vi "CLC_GEN3_L2_InPhaseCal_mW_BaseOnly_L&S.vi"() -> ()   [LabVIEW 2023, in "Clover_Cell.lvlib"]
uses:
  Clover_Cell.lvlib
  lib/ELTA/ELTA.lvlib
  lib/R_S/R_S.lvlib
  lib/LitePoints/LitePoints.lvlib
panel:
  in  "Base_Gain":i32
  in  "Base_Phase":i32
  in  "Base_Ch":i32
  in  "Daul_Ch_Phase_Sweep":bool
  in  "SweepSwitch?":u16(ring) items=["NoSweep(Single)", "Sweep"]
  in  "SweepMode":u16(ring) items=["Phase", "Gain"]
  in  "Method":u16(ring)=1 items=["dBm"=1, "mW"=2]
  in  "Polarity":u16(ring) items=["H", "V"]
  in  "Spectrum_VISA":refnum<visa-resource-name>="TCPIP0::192.168.100.230::inst0::INSTR"
  in  "CenterFreq(GHz)":dbl=28.0
  in  "AvgTimes":i32=3
  in  "Single_Ch_Phase_Sweep":bool
  in  "TRXmode":u16(ring)=1 items=["Rx"=2, "Tx"=1]
  out "GainStep":i32=63
  out "PhaseStep":i32=63
  out "Channel":i32=63
  out "Total mW":dbl format="%.7f"
  out "Total dBm":dbl format="%.7f"
  out "Ref. mW":dbl format="%.7f"
  out "Ref. dBm":dbl format="%.7f"
  out "Main mW":dbl format="%.7f"
  out "Main dBm":dbl format="%.7f"
  out "Data":dbl[][](array[numeric])
  out "FileNAME_Single":string
  out "Spectrum Analyzer":dbl[](graph)
  out "CurrentData":dbl[](array[numeric])
  out "Duration":dbl
  out "TotalTime":dbl format="%.2f"
  out "StopTime":timestamp=timestamp(3663835912.033212 s since 1904-01-01)
  out "FileNAME_Dual":string
  out "StartTime":timestamp=timestamp(3663835741.875155 s since 1904-01-01)
  out "TX/RX":u16=1
  out "error out":errorcluster
  out "output cluster":T1={"address"="192.168.100.111", "remote port or service name"=5025, "timeout ms (60000)"=10000}
  out "Operating \nChannel(s)":bool[][](array[boolean])
  out "OK?":bool
  # "TMYTEK_CLC_JIO_One_Panel_Phase_Calibration"
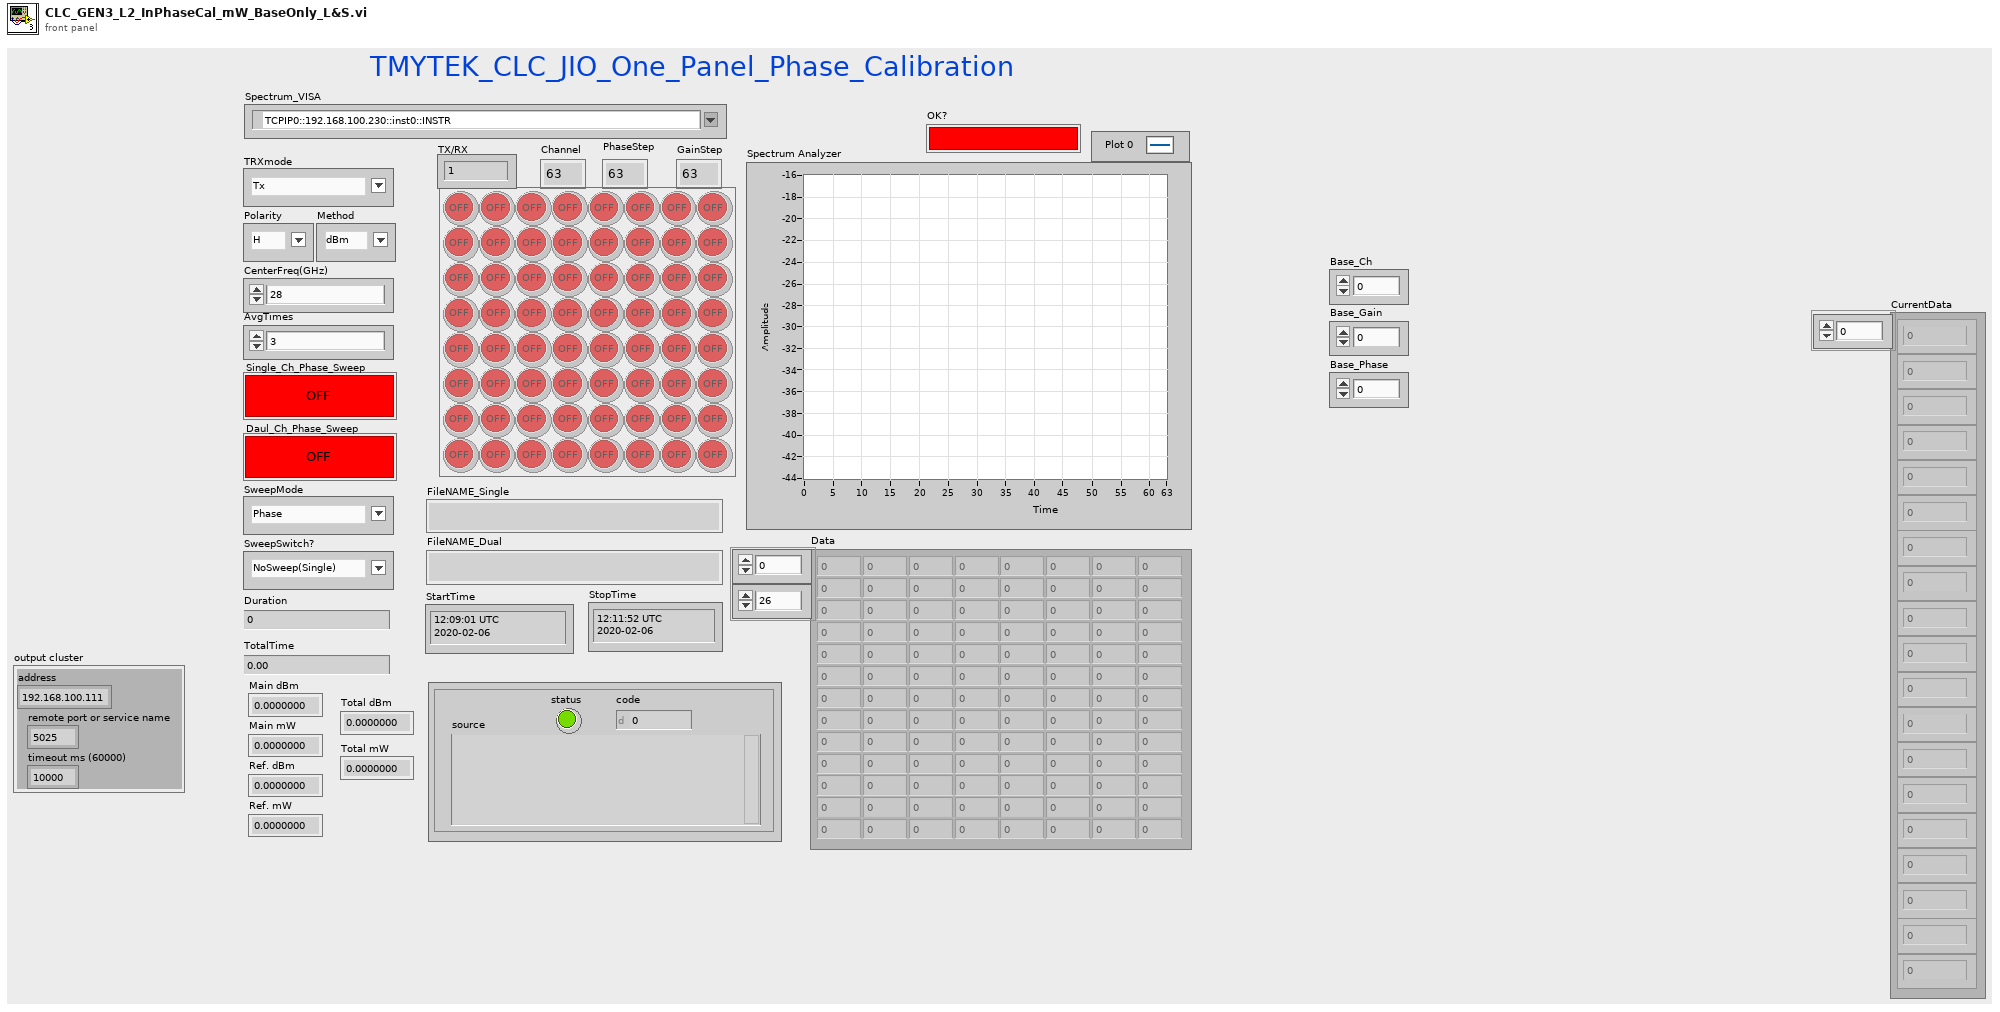
[diagram p1: front panel]
types:
  T1 = cluster{"address":string, "remote port or service name":u16, "timeout ms (60000)":i32}
  T2 = cluster{"Mode":u16, "Polarity":u16, "CH_ON/OFF":u16, "Channel":i32, "Gain":i32, "Phase":i32}
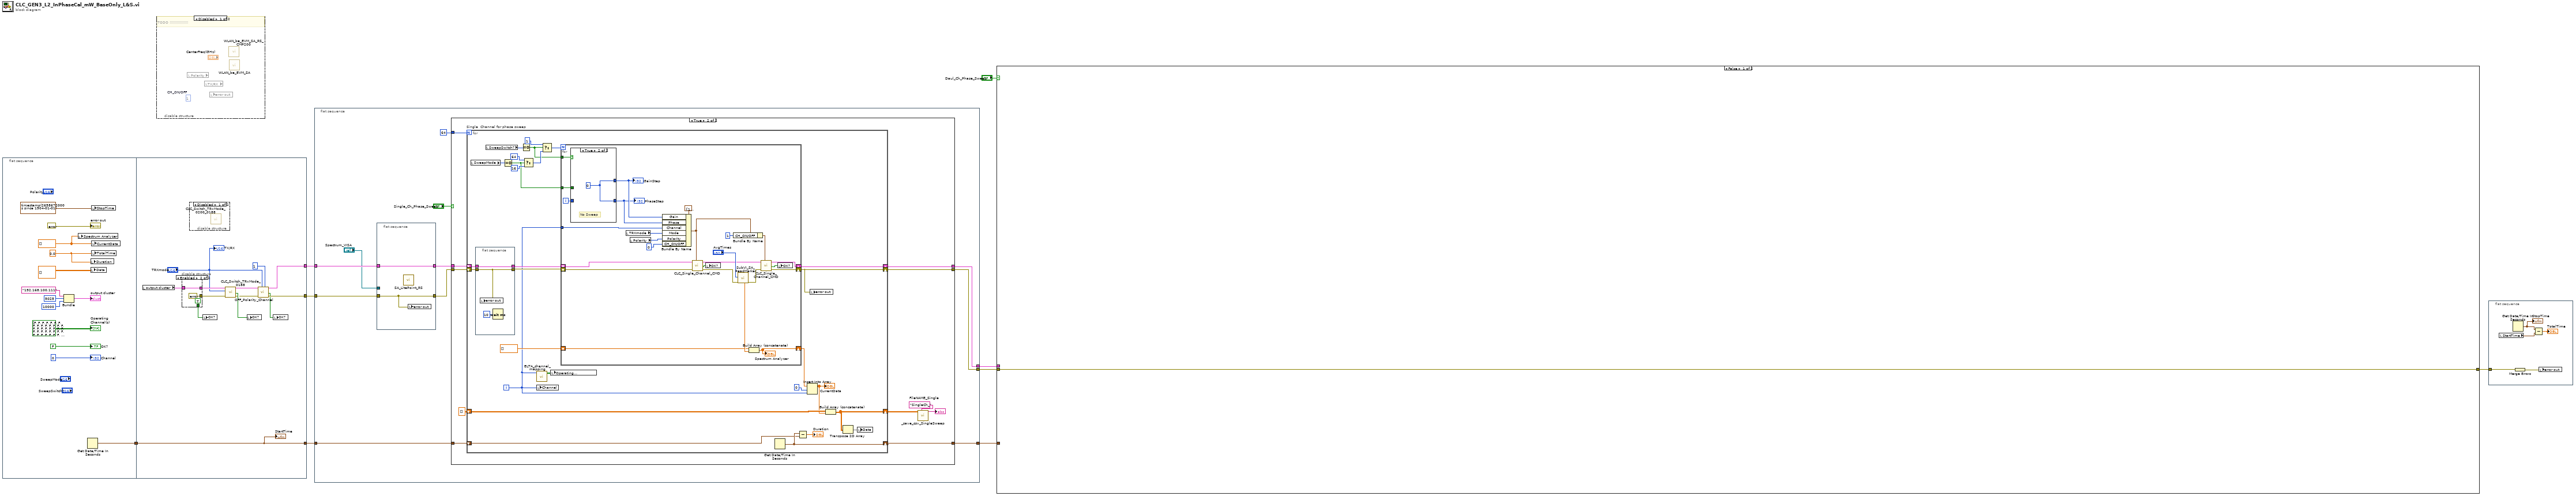
[diagram p0: block diagram]
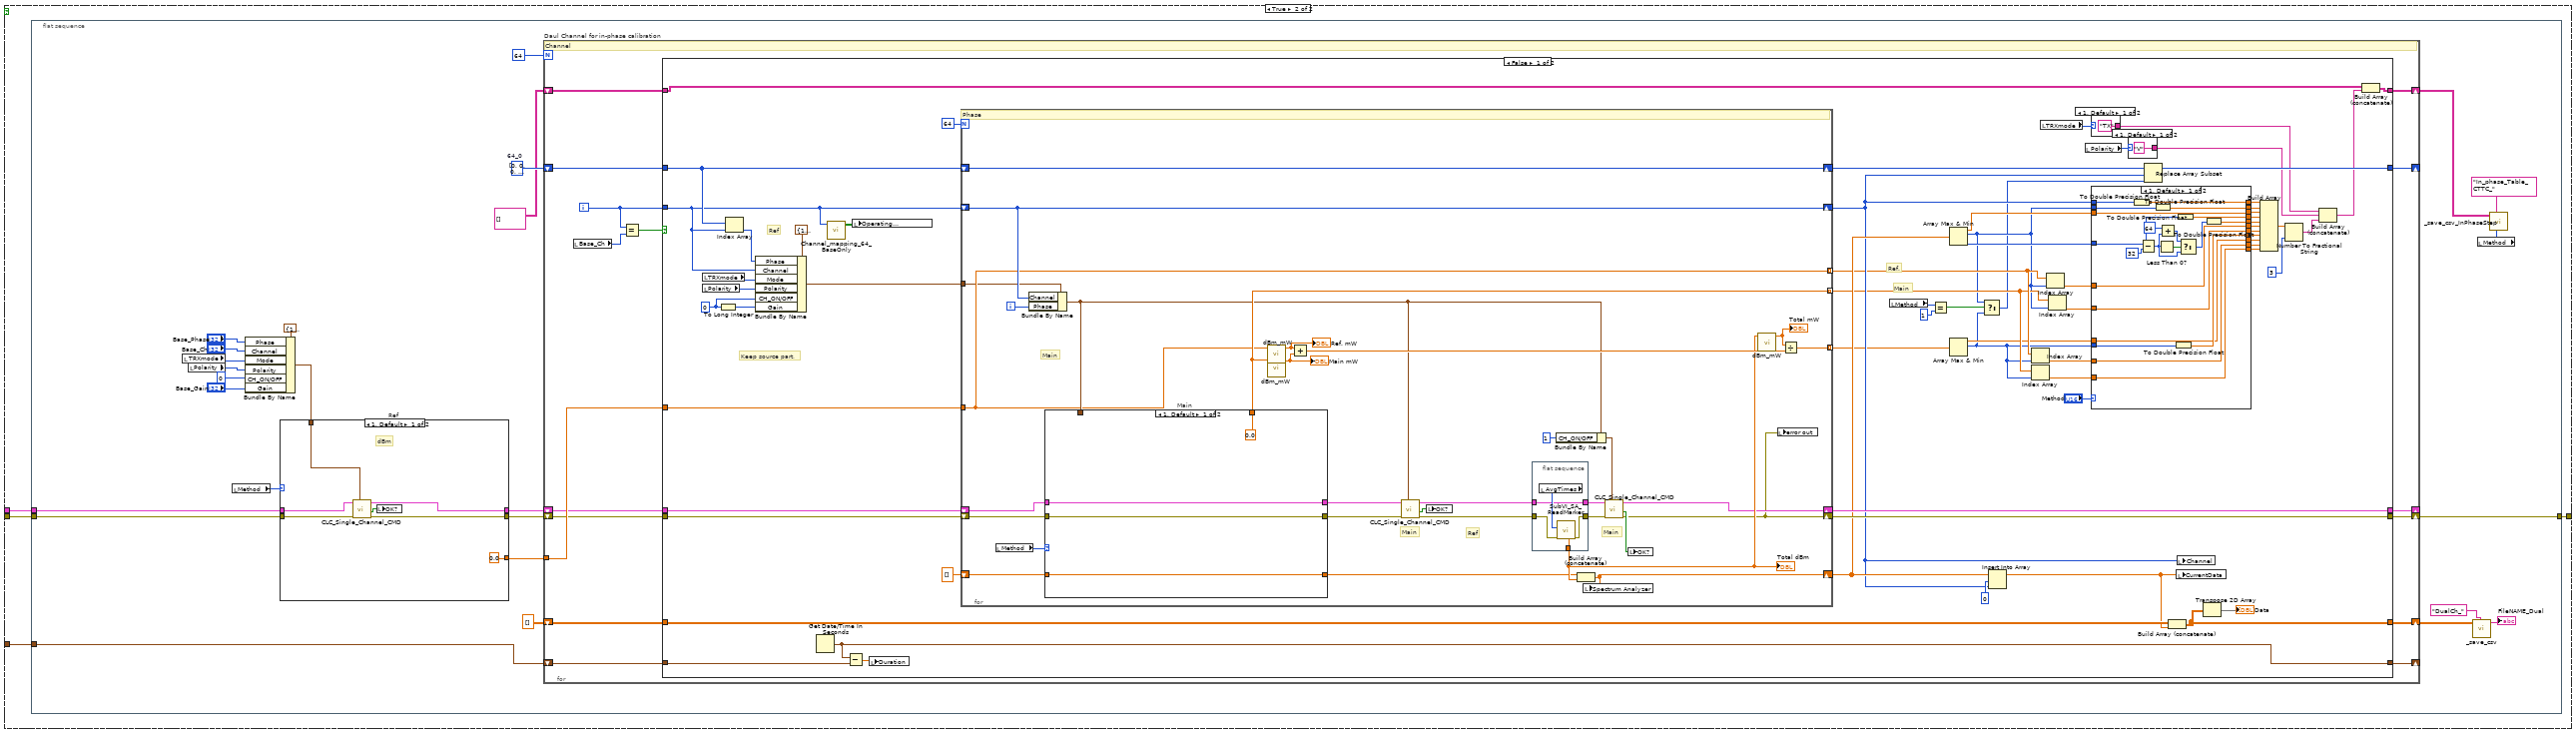
[diagram p3: hidden frame]
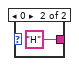
[diagram p4: hidden frame]
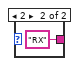
[diagram p5: hidden frame]
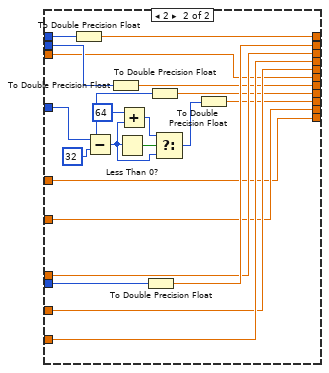
[diagram p6: hidden frame]
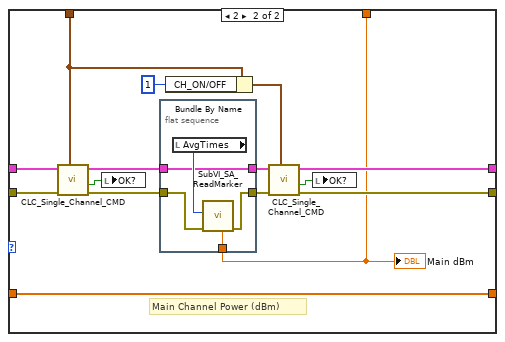
[diagram p7: hidden frame]
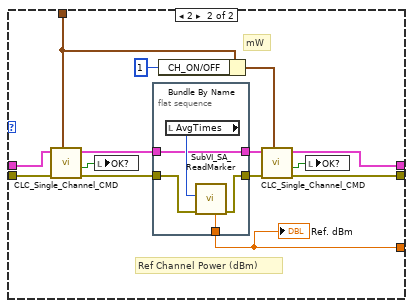
[diagram p9: hidden frame]
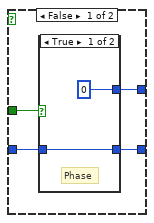
[diagram p11: hidden frame]
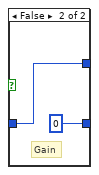
[diagram p12: hidden frame]
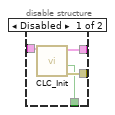
[diagram p14: hidden frame]
diagram:
  n1 = flat-sequence {
    tunnel: [w10] -> w9
    tunnel: w9 -> [w25]
    tunnel: [w27] -> w2
    tunnel: [w30] -> w3
    tunnel: [w25] -> w8
    frame #0 {
      w14 = dbl[] []
      w17 = 0.0 ("TotalTime")
      n2 = Bundle("address"="192.168.100.111", "remote port or service name"=u16 5025, "timeout ms (60000)"=10000) -> (→"output cluster":T1)  [unwired: 1 in]
      n3 = local write "Spectrum Analyzer"(w14) -> ()
      n4 = Get Date/Time In Seconds() -> (seconds since 1Jan1904=w10:timestamp)
      n5 = local write "Duration"(w17) -> ()
      n6 = local write "Data"(dbl[][] []) -> ()
      n7 = local write "StopTime"(timestamp(2658672000.001 s since 1904-01-01) ("StopTime")) -> ()
      n8 = local write "CurrentData"(w14) -> ()
      n9 = local write "TotalTime"(w17) -> ()
      "error out" <- errorcluster {"status"=FALSE, "code"=0, "source"=""} ("error out")
      "Operating \nChannel(s)" <- bool[][] [[FALSE, FALSE, FALSE, FALSE, FALSE, FALSE, FALSE, FALSE], [FALSE, FALSE, FALSE, FALSE, FALSE, FALSE, FALSE, FALSE], [FALSE, FALSE, FALSE, FALSE, FALSE, FALSE, FALSE, FALSE], [FALSE, FALSE, FALSE, FALSE, FALSE, FALSE, FALSE, FALSE], [FALSE, FALSE, FALSE, FALSE, FALSE, FALSE, FALSE, FALSE], [FALSE, FALSE, FALSE, FALSE, FALSE, FALSE, FALSE, FALSE], [FALSE, FALSE, FALSE, FALSE, FALSE, FALSE, FALSE, FALSE], [FALSE, FALSE, FALSE, FALSE, FALSE, FALSE, FALSE, FALSE]] ("Operating \nChannel(s)")
      "Channel" <- 0 ("Channel")
      "OK?" <- FALSE ("OK?")
    }
    frame #1 {
      n10 = local read "output cluster"() -> (w35:T1)
      n11 = disable-structure shown="Enabled" {
        disable-tunnel: w35 -> [w39 w42]
        disable-tunnel: [w38 w42] -> w34
        disable-tunnel: [w37 errorcluster {"status"=FALSE, "code"=0, "source"=""} ("error in (no error)")] -> w32
        disable-tunnel: [w36 TRUE ("OK?")] -> w26
        frame Disabled {
          n12 = call "CLC_Init.vi"("TCPIPin"=w39) -> ("error out"=w37:errorcluster, "Status"=w36:bool, "TCPIPin 2"=w38:T1)  [unwired: 8 in]
        }
        frame Enabled {
        }
      }
      n13 = disable-structure shown="Disabled" {
        frame Disabled {
          n14 = call "CLC_Switch_TRxMode_0200_0188.vi"() -> ()  [unwired: 9 in, 3 out]
        }
        frame Enabled {
        }
      }
      n15 = local write "OK?"(w26) -> ()
      n16 = call "CLC_Switch_TRxMode_0188.vi"("error in (no error)"=w32, "Text Ring"="TRXmode", "TCPIPin"=w34) -> ("error out"=w31:errorcluster, "OK?"=w33:bool, "TCPIPin 2"=w29:T1)  [unwired: 6 in]
      n17 = local write "OK?"(w33) -> ()
      n18 = call "OFF_Polarity_Channel.vi"("CH_ON:0/OFF:1"=u16 1, "Mode"="TRXmode", "error in"=w31, "TCPIPin"=w29) -> ("error out"=w30:errorcluster, "OK?"=w28:bool, "TCPIPout"=w27:T1)  [unwired: 5 in]
      n19 = local write "OK?"(w28) -> ()
      "StartTime" <- w25
      "TX/RX" <- "TRXmode"
    }
  }
  n20 = disable-structure shown="Disabled" {
    frame Disabled {
      (unwired) u16 1  # CH_ON/OFF
      # "TODO !!!!!!!!!!!!!!!!"
      n21 = local read "Polarity"() -> ()  [unwired: 1 out]
      n22 = local read "TX/RX"() -> ()  [unwired: 1 out]
      n23 = local read "error out"() -> ()  [unwired: 1 in]
      n24 = call "WLAN_be_EVM_SA_RS_CMP200.vi"() -> ()  [unwired: 8 in, 4 out]
      n25 = call "WLAN_be_EVM_SA.vi"() -> ()  [unwired: 8 in, 4 out]
    }
    frame Enabled {
    }
  }
  n26 = flat-sequence {
    tunnel: w8 -> [w52]
    tunnel: [w51] -> w7
    tunnel: [w50] -> w6
    tunnel: [w49] -> w4
    tunnel: w3 -> [w48]
    tunnel: w2 -> [w46]
    frame #0 {
      n27 = flat-sequence {
        tunnel: w48 -> [w134]
        tunnel: [w134] -> w47
        tunnel: w46 -> [w133]
        tunnel: "Spectrum_VISA" -> [_]
        tunnel: [w133] -> w44
        frame #0 {
          n28 = call "SA_LitePoint_RS.vi"() -> ()  [unwired: 12 in]
          n29 = local write "error out"(w134) -> ()
        }
      }
      n30 = case shown="True" "Single_Ch_Phase_Sweep" {
        tunnel: 64 -> [_ w67]
        tunnel: w52 -> [w54 w66]
        tunnel: [w55 w65] -> w51
        tunnel: [w56 w64] -> w50
        tunnel: [w54 w63] -> w49
        tunnel: w47 -> [w55 w62]
        tunnel: w44 -> [w56 w61]
        frame False {
        }
        frame True {
          n31 = for "Single  Channel for phase sweep" {
            N: w67 -> [_]
            shift-right: [w94] -> w64
            shift-left: w61 -> [w81]
            shift-right: [w90] -> w65
            shift-left: w62 -> [w83]
            shift-right: [w88] -> w58
            shift-left: dbl[][] [] -> [w89]
            shift-right: [w92] -> w63
            shift-left: w66 -> [w91]
            i -> [w68]
            n32 = local read "SweepMode"() -> (w77:u16)
            n33 = flat-sequence {
              tunnel: [w95] -> w80
              tunnel: w83 -> [w96]
              tunnel: [w96] -> w82
              tunnel: w81 -> [w95]
              frame #0 {
                n34 = local write "error out"(w96) -> ()
                n35 = Wait (ms)(milliseconds to wait=u32 10) -> ()  [unwired: 1 out]
              }
            }
            n36 = local read "SweepSwitch?"() -> (w76:u16)
            n37 = Equal To 0?(x=w77) -> (x = 0?=w69:bool)
            n38 = Equal To 0?(x=w76) -> (x = 0?=w70:bool)
            n39 = Select(t=64, s=w69, f=16) -> (s? t:f=w71:i32)
            n40 = local write "Channel"(w68) -> ()
            n41 = call "ELTA_channel_mapping.vi"("Ch_1_ref"=w68) -> ("Operating \nChannel(s)"=w78:bool[][])  [unwired: 10 in]
            n42 = Select(t=1, s=w70, f=w71) -> (s? t:f=w74:i32)
            n43 = local write "Operating \nChannel(s)"(w78) -> ()
            n44 = for {
              N: w74 -> [_]
              shift-right: [w107] -> w94
              shift-left: w80 -> [w117]
              shift-right: [w109] -> w90
              shift-left: w82 -> [w119]
              shift-right: [w120] -> w87
              shift-left: dbl[] [] -> [w121]
              tunnel: w68 -> [w114]
              tunnel: w70 -> [w102]
              tunnel: w69 -> [w99]
              i -> [w98]
              n45 = case shown="True" w102 {
                tunnel: [w124 w132] -> w101
                tunnel: [w125 w132] -> w100
                tunnel: w99 -> [w127 _]
                tunnel: w98 -> [w126 _]
                frame False {
                  n46 = case shown="True" w127 {
                    tunnel: w126 -> [w129 w130]
                    tunnel: [w129 0] -> w125
                    tunnel: [0 w130] -> w124
                    frame True {
                      # "Phase"
                    }
                    frame False {
                      # "Gain"
                    }
                  }
                }
                frame True {
                  w132 = 0
                  # "No Sweep"
                }
              }
              "PhaseStep" <- w100
              "GainStep" <- w101
              n47 = local read "TRXmode"() -> (w113:u16)
              n48 = local read "Polarity"() -> (w112:u16)
              n49 = Bundle By Name(cluster=T2 {"Mode"=1, "Polarity"=1, "CH_ON/OFF"=1, "Channel"=0, "Gain"=0, "Phase"=0} ("Channel params"), "Gain"=w101, "Phase"=w100, "Channel"=w114, "Mode"=w113, "Polarity"=w112, "CH_ON/OFF"=u16 0) -> (w106:T2)
              n50 = call "CLC_Single_Channel_CMD.vi"("Channel params"=w106, "error in"=w119, "TCPIPin"=w117) -> ("error out"=w118:errorcluster, "OK?"=w115:bool, "TCPIPout"=w108:T1)  [unwired: 6 in]
              n51 = local write "OK?"(w115) -> ()
              n52 = Bundle By Name(cluster=w106, "CH_ON/OFF"=u16 1) -> (w104:T2)
              n53 = call "SubVI_SA_ReadMarker.vi"("error in (no error)"=w118, "AvgTimes"="AvgTimes") -> ("error out"=w110:errorcluster, "Marker Power"=w122:dbl)  [unwired: 6 in, 2 out]
              n54 = Build Array (concatenate)(w121, w122) -> (w120:dbl[])
              "Spectrum Analyzer" <- w120
              n55 = call "CLC_Single_Channel_CMD.vi"("Channel params"=w104, "error in"=w110, "TCPIPin"=w108) -> ("error out"=w109:errorcluster, "OK?"=w103:bool, "TCPIPout"=w107:T1)  [unwired: 6 in]
              n56 = local write "OK?"(w103) -> ()
            }
            n57 = Get Date/Time In Seconds() -> (seconds since 1Jan1904=w92:timestamp)
            n58 = Subtract(x=w92, y=w91) -> (x-y=→"Duration":dbl)
            n59 = Insert Into Array(array=w87, index=0, new element=w68) -> (w85:dbl[])
            "CurrentData" <- w85
            n60 = local write "error out"(w90) -> ()
            n61 = Build Array (concatenate)(w89, w85) -> (w88:dbl[][])
            n62 = Transpose 2D Array(2D array=w88) -> (transposed array=w79:dbl[][])
            n63 = local write "Data"(w79) -> ()
          }
          n64 = call "_save_csv_SingleSweep.vi"("delimiter (\\t)"="SingleCh_" ("delimiter (\\t)"), "Data"=w58) -> ("FileName"=→"FileNAME_Single":string)  [unwired: 9 in]
        }
      }
    }
  }
  n65 = case shown="False" "Daul_Ch_Phase_Sweep" {
    tunnel: w7 -> [w135 w139]
    tunnel: w6 -> [_ w138]
    tunnel: [w135 w137] -> w5
    tunnel: w4 -> [_ w136]
    frame False {
    }
    frame True {
      n66 = flat-sequence {
        tunnel: w139 -> [w150]
        tunnel: w138 -> [w151]
        tunnel: [w164] -> w137
        tunnel: w136 -> [w163]
        frame #0 {
          w161 = i32[] [0, 0, 0, 0, 0, 0, 0, 0, 0, 0, 0, 0, 0, 0, 0, 0, 0, 0, 0, 0, 0, 0, 0, 0, 0, 0, 0, 0, 0, 0, 0, 0, 0, 0, 0, 0, 0, 0, 0, 0, 0, 0, 0, 0, 0, 0, 0, 0, 0, 0, 0, 0, 0, 0, 0, 0, 0, 0, 0, 0, 0, 0, 0, 0]  # 64_0
          n67 = local read "TRXmode"() -> (w147:u16)
          n68 = local read "Polarity"() -> (w148:u16)
          n69 = local read "Method"() -> (w155:u16)
          n70 = Bundle By Name(cluster=T2 {"Mode"=1, "Polarity"=1, "CH_ON/OFF"=1, "Channel"=0, "Gain"=0, "Phase"=0} ("Channel params"), "Phase"="Base_Phase", "Channel"="Base_Ch", "Mode"=w147, "Polarity"=w148, "CH_ON/OFF"=u16 0, "Gain"="Base_Gain") -> (w145:T2)
          n71 = case "Ref" shown="1, Default" w155 {
            tunnel: w150 -> [w363 w373]
            tunnel: [w366 w372] -> w153
            tunnel: w151 -> [w364 w371]
            tunnel: [w365 w370] -> w152
            tunnel: [0.0 ("Marker Response") w369] -> w154
            tunnel: w145 -> [w362 w368]
            frame 1, Default {
              # "dBm"
              n72 = call "CLC_Single_Channel_CMD.vi"("Channel params"=w362, "error in"=w363, "TCPIPin"=w364) -> ("error out"=w366:errorcluster, "OK?"=w361:bool, "TCPIPout"=w365:T1)  [unwired: 6 in]
              n73 = local write "OK?"(w361) -> ()
            }
            frame 2 {
              # "mW"
              # "Ref Channel Power (dBm)"
              n74 = call "CLC_Single_Channel_CMD.vi"("Channel params"=w368, "error in"=w373, "TCPIPin"=w371) -> ("error out"=w380:errorcluster, "OK?"=w381:bool, "TCPIPout"=w379:T1)  [unwired: 6 in]
              n75 = local write "OK?"(w381) -> ()
              n76 = flat-sequence {
                tunnel: [w385] -> w369
                tunnel: w380 -> [w384]
                tunnel: [w383] -> w375
                tunnel: w379 -> [w383]
                tunnel: [w382] -> w376
                frame #0 {
                  n77 = local read "AvgTimes"() -> (w386:i32)
                  n78 = call "SubVI_SA_ReadMarker.vi"("error in (no error)"=w384, "AvgTimes"=w386) -> ("error out"=w382:errorcluster, "Marker Power"=w385:dbl)  [unwired: 6 in, 2 out]
                }
              }
              n79 = Bundle By Name(cluster=w368, "CH_ON/OFF"=u16 1) -> (w377:T2)
              n80 = call "CLC_Single_Channel_CMD.vi"("Channel params"=w377, "error in"=w376, "TCPIPin"=w375) -> ("error out"=w372:errorcluster, "OK?"=w378:bool, "TCPIPout"=w370:T1)  [unwired: 6 in]
              n81 = local write "OK?"(w378) -> ()
              "Ref. dBm" <- w369
            }
          }
          n82 = for "Daul Channel for in-phase calibration" {
            N: 64 -> [_]
            shift-right: [w181] -> _
            shift-left: w152 -> [w171]
            shift-right: [w180] -> w164
            shift-left: w153 -> [w170]
            shift-right: [w176] -> w157
            shift-left: dbl[][] [] -> [w177]
            shift-right: [w179] -> _
            shift-left: w163 -> [w178]
            shift-right: [w175] -> _
            shift-left: w161 -> [w174]
            tunnel: w154 -> [w172]
            shift-right: [w173] -> w141
            shift-left: string[][] [] -> [w166]
            i -> [w168]
            # "Channel"
            n83 = local read "Base_Ch"() -> (w169:i32)
            n84 = Equal?(x=w168, y=w169) -> (x = y?=w167:bool)
            n85 = case shown="False" w167 {
              tunnel: [w248 w359] -> w181
              tunnel: [w246 w358] -> w180
              tunnel: [w245 w356] -> w179
              tunnel: w178 -> [w244 w356]
              tunnel: w177 -> [w242 w357]
              tunnel: [w241 w357] -> w176
              tunnel: [w235 w360] -> w175
              tunnel: w174 -> [w217 w360]
              tunnel: [w183 w355] -> w173
              tunnel: w172 -> [w188 _]
              tunnel: w171 -> [w187 w359]
              tunnel: w170 -> [w186 w358]
              tunnel: w168 -> [w185 _]
              tunnel: w166 -> [w182 w355]
              frame False {
                w219 = u16 0 ("CH_ON/OFF")
                # "Keep source part,"
                # "Main"
                # "Ref."
                # "Ref"
                n86 = local read "TRXmode"() -> (w221:u16)
                n87 = local read "Polarity"() -> (w220:u16)
                n88 = To Long Integer(number=w219) -> (32bit integer=w218:i32)
                n89 = Index Array(array=w217, index=w185) -> (element=w216:i32)
                n90 = Bundle By Name(cluster=T2 {"Mode"=1, "Polarity"=1, "CH_ON/OFF"=1, "Channel"=0, "Gain"=0, "Phase"=0} ("Channel params"), "Phase"=w216, "Channel"=w185, "Mode"=w221, "Polarity"=w220, "CH_ON/OFF"=w219, "Gain"=w218) -> (w184:T2)
                n91 = Get Date/Time In Seconds() -> (seconds since 1Jan1904=w245:timestamp)
                n92 = call "Channel_mapping_64_BaseOnly.vi"("Channel IN"=w185) -> ("Operating \nChannel(s)"=w223:bool[][])  [unwired: 10 in]
                n93 = Subtract(x=w245, y=w244) -> (x-y=w243:dbl)
                n94 = local write "Operating \nChannel(s)"(w223) -> ()
                n95 = local write "Duration"(w243) -> ()
                n96 = for {
                  N: 64 -> [_]
                  shift-right: [w297] -> w248
                  shift-left: w187 -> [w307]
                  shift-right: [w296] -> w246
                  shift-left: w186 -> [w318]
                  shift-right: [w320] -> w236
                  shift-left: dbl[] [] -> [w309]
                  shift-right: [w324] -> w234
                  shift-left: w217 -> [w324]
                  shift-right: [w303] -> w233
                  shift-left: w185 -> [w303]
                  tunnel: [w300] -> w226 mode=indexing
                  tunnel: [w313] -> w225 mode=indexing
                  tunnel: [w314] -> w232 mode=indexing
                  tunnel: w188 -> [w300]
                  tunnel: w184 -> [w295]
                  i -> [w304]
                  # "Main"
                  # "Main"
                  # "Ref"
                  # "Main"
                  # "Phase"
                  n97 = local read "Method"() -> (w310:u16)
                  n98 = Bundle By Name(cluster=w295, "Channel"=w303, "Phase"=w304) -> (w302:T2)
                  n99 = case "Main" shown="1, Default" w310 {
                    tunnel: w318 -> [w327 w332]
                    tunnel: w307 -> [w328 w333]
                    tunnel: [w328 w336] -> w317
                    tunnel: [w327 w335] -> w316
                    tunnel: w302 -> [_ w334]
                    tunnel: [0.0 ("Marker Response") w330] -> w313
                    tunnel: w309 -> [w326 w331]
                    tunnel: [w326 w331] -> w308
                    frame 1, Default {
                    }
                    frame 2 {
                      # "Main Channel Power (dBm)"
                      n100 = call "CLC_Single_Channel_CMD.vi"("Channel params"=w334, "error in"=w332, "TCPIPin"=w333) -> ("error out"=w338:errorcluster, "OK?"=w337:bool, "TCPIPout"=w339:T1)  [unwired: 6 in]
                      n101 = local write "OK?"(w337) -> ()
                      n102 = flat-sequence {
                        tunnel: [w348] -> w330
                        tunnel: w338 -> [w347]
                        tunnel: [w346] -> w344
                        tunnel: w339 -> [w346]
                        tunnel: [w345] -> w343
                        frame #0 {
                          n103 = local read "AvgTimes"() -> (w349:i32)
                          n104 = call "SubVI_SA_ReadMarker.vi"("error in (no error)"=w347, "AvgTimes"=w349) -> ("error out"=w345:errorcluster, "Marker Power"=w348:dbl)  [unwired: 6 in, 2 out]
                        }
                      }
                      n105 = Bundle By Name(cluster=w334, "CH_ON/OFF"=u16 1) -> (w342:T2)
                      n106 = call "CLC_Single_Channel_CMD.vi"("Channel params"=w342, "error in"=w343, "TCPIPin"=w344) -> ("error out"=w335:errorcluster, "OK?"=w340:bool, "TCPIPout"=w336:T1)  [unwired: 6 in]
                      n107 = local write "OK?"(w340) -> ()
                      "Main dBm" <- w330
                    }
                  }
                  n108 = call "dBm_mW.vi"("dBm"=w300) -> ("mW"=w306:dbl)  [unwired: 10 in]
                  "Ref. mW" <- w306
                  n109 = call "dBm_mW.vi"("dBm"=w313) -> ("mW"=w305:dbl)  [unwired: 10 in]
                  "Main mW" <- w305
                  n110 = Add(x=w306, y=w305) -> (x+y=w315:dbl)
                  n111 = call "CLC_Single_Channel_CMD.vi"("Channel params"=w302, "error in"=w316, "TCPIPin"=w317) -> ("error out"=w298:errorcluster, "OK?"=w325:bool, "TCPIPout"=w299:T1)  [unwired: 6 in]
                  n112 = local write "OK?"(w325) -> ()
                  n113 = flat-sequence {
                    tunnel: [w353] -> w312
                    tunnel: w298 -> [w352]
                    tunnel: [w351] -> w323
                    tunnel: w299 -> [w351]
                    tunnel: [w350] -> w319
                    frame #0 {
                      n114 = local read "AvgTimes"() -> (w354:i32)
                      n115 = call "SubVI_SA_ReadMarker.vi"("error in (no error)"=w352, "AvgTimes"=w354) -> ("error out"=w350:errorcluster, "Marker Power"=w353:dbl)  [unwired: 6 in, 2 out]
                    }
                  }
                  n116 = Bundle By Name(cluster=w302, "CH_ON/OFF"=u16 1) -> (w321:T2)
                  n117 = Build Array (concatenate)(w308, w312) -> (w320:dbl[])
                  n118 = local write "Spectrum Analyzer"(w320) -> ()
                  n119 = call "CLC_Single_Channel_CMD.vi"("Channel params"=w321, "error in"=w319, "TCPIPin"=w323) -> ("error out"=w296:errorcluster, "OK?"=w322:bool, "TCPIPout"=w297:T1)  [unwired: 6 in]
                  n120 = local write "OK?"(w322) -> ()
                  n121 = call "dBm_mW.vi"("dBm"=w312) -> ("mW"=w311:dbl)  [unwired: 10 in]
                  "Total mW" <- w311
                  n122 = local write "error out"(w296) -> ()
                  n123 = Divide(x=w311, y=w315) -> (x/y=w314:dbl)
                  "Total dBm" <- w312
                }
                n124 = local read "Method"() -> (w203:u16)
                n125 = Equal?(x=w203, y=u16 1) -> (x = y?=w201:bool)
                n126 = Array Max & Min(array=w236) -> (max value=w213:dbl, max index (indices)=w200:i32, min index (indices)=w224:i32)  [unwired: 1 out]
                n127 = Array Max & Min(array=w232) -> (max value=w207:dbl, max index (indices)=w199:i32)  [unwired: 2 out]
                n128 = Select(t=w200, s=w201, f=w199) -> (s? t:f=w198:i32)
                n129 = Insert Into Array(array=w236, index=0, new element=w233) -> (w237:dbl[])
                n130 = Index Array(array=w226, index=w199) -> (element=w206:dbl)
                n131 = Index Array(array=w225, index=w199) -> (element=w205:dbl)
                n132 = local read "TRXmode"() -> (w194:u16)
                n133 = Index Array(array=w226, index=w200) -> (element=w211:dbl)
                n134 = Index Array(array=w225, index=w200) -> (element=w210:dbl)
                n135 = local read "Polarity"() -> (w193:u16)
                n136 = case shown="1, Default" w194 {
                  tunnel: ["TX" "RX"] -> w190
                  frame 1, Default {
                  }
                  frame 2 {
                  }
                }
                n137 = case shown="1, Default" "Method" {
                  tunnel: w233 -> [w267 w288]
                  tunnel: [w253 w282] -> w231
                  tunnel: [w266 w281] -> w230
                  tunnel: [w265 w280] -> w229
                  tunnel: [w264 w284] -> w228
                  tunnel: [w263 w277] -> w227
                  tunnel: w224 -> [w262 w287]
                  tunnel: w199 -> [w261 w286]
                  tunnel: w200 -> [w260 w285]
                  tunnel: w213 -> [w253 w279]
                  tunnel: [w254 w283] -> w214
                  tunnel: [w259 w279] -> w212
                  tunnel: w211 -> [w259 w274]
                  tunnel: w210 -> [w258 w275]
                  tunnel: [w258 w278] -> w209
                  tunnel: [w257 w276] -> w208
                  tunnel: w207 -> [w257 w282]
                  tunnel: w206 -> [w256 w280]
                  tunnel: w205 -> [w255 w281]
                  tunnel: [w255 w274] -> w204
                  tunnel: [w256 w275] -> w197
                  frame 1, Default {
                    n138 = To Double Precision Float(number=w267) -> (double precision float=w264:dbl)
                    n139 = Subtract(x=w262, y=32) -> (x-y=w269:i32)
                    n140 = To Double Precision Float(number=w260) -> (double precision float=w254:dbl)
                    n141 = Less Than 0?(x=w269) -> (x < 0?=w272:bool)
                    n142 = Add(x=64, y=w269) -> (x+y=w270:i32)
                    n143 = To Double Precision Float(number=w261) -> (double precision float=w263:dbl)
                    n144 = To Double Precision Float(number=w262) -> (double precision float=w266:dbl)
                    n145 = Select(t=w270, s=w272, f=w269) -> (s? t:f=w268:i32)
                    n146 = To Double Precision Float(number=w268) -> (double precision float=w265:dbl)
                  }
                  frame 2 {
                    n147 = To Double Precision Float(number=w288) -> (double precision float=w284:dbl)
                    n148 = Subtract(x=w287, y=32) -> (x-y=w290:i32)
                    n149 = To Double Precision Float(number=w285) -> (double precision float=w278:dbl)
                    n150 = Less Than 0?(x=w290) -> (x < 0?=w293:bool)
                    n151 = Add(x=64, y=w290) -> (x+y=w291:i32)
                    n152 = To Double Precision Float(number=w286) -> (double precision float=w283:dbl)
                    n153 = To Double Precision Float(number=w287) -> (double precision float=w277:dbl)
                    n154 = Select(t=w291, s=w293, f=w290) -> (s? t:f=w289:i32)
                    n155 = To Double Precision Float(number=w289) -> (double precision float=w276:dbl)
                  }
                }
                n156 = case shown="1, Default" w193 {
                  tunnel: ["V" "H"] -> w191
                  frame 1, Default {
                  }
                  frame 0 {
                  }
                }
                n157 = Replace Array Subset(array=w234, new element=w198, index=w233) -> (w235:i32[])
                n158 = Build Array (concatenate)(w242, w237) -> (w241:dbl[][])
                n159 = local write "CurrentData"(w237) -> ()
                n160 = local write "Channel"(w233) -> ()
                n161 = Transpose 2D Array(2D array=w241) -> (transposed array=→"Data":dbl[][])
                n162 = Build Array(w228, w214, w231, w230, w229, w212, w209, w227, w208, w197, w204) -> (w195:dbl[])
                n163 = Number To Fractional String(number=w195, precision (6)=i16 3) -> (F-format string=w192:string[])  [unwired: 2 in]
                n164 = Build Array (concatenate)(w190, w191, w192) -> (w189:string[])
                n165 = Build Array (concatenate)(w182, w189) -> (w183:string[][])
              }
              frame True {
              }
            }
          }
          n166 = call "_save_csv.vi"("delimiter (\\t)"="DualCh_" ("delimiter (\\t)"), "Data"=w157) -> ("FileName"=→"FileNAME_Dual":string)  [unwired: 9 in]
          n167 = local read "Method"() -> (w156:u16)
          n168 = call "_save_csv_InPhaseStep.vi"("Method"=w156, "delimiter (\\t)"="In_phase_Table_CTTC_" ("delimiter (\\t)"), "dataInput"=w141) -> ()  [unwired: 8 in, 1 out]
        }
      }
    }
  }
  n169 = flat-sequence {
    tunnel: w5 -> [w387]
    frame #0 {
      n170 = local read "StartTime"() -> (w388:timestamp)
      n171 = Get Date/Time In Seconds() -> (seconds since 1Jan1904=w389:timestamp)
      "StopTime" <- w389
      n172 = Merge Errors(w387) -> (w391:errorcluster)
      n173 = Subtract(x=w389, y=w388) -> (x-y=→"TotalTime":dbl)
      n174 = local write "error out"(w391) -> ()
    }
  }
